vi "Handle Error.vi"(8 "error in (no error)":errorcluster caption="错误输入（无错误）", 11 "ErrorHanlder in":refnum<class "ErrorHanlder.lvclass"> caption="操作者输入") -> (0 "error out":errorcluster caption="错误输出", 2 "stop actor?":bool=TRUE caption="停止操作者？", 3 "ErrorHanlder out":refnum<class "ErrorHanlder.lvclass"> caption="操作者输出")   [LabVIEW 2019, in "ErrorHanlder.lvlib" / "ErrorHanlder.lvclass"]
doc: "(<B>Filename</B>: Actor Framework.lvlib:Actor.lvclass:Handle Error.vi)\n\nDefines how the actor handles an error that occurred while processing a message.默认情况下，该方法不执行任何操作，仅停止操作者。"
uses:
  ErrorHanlder.lvclass
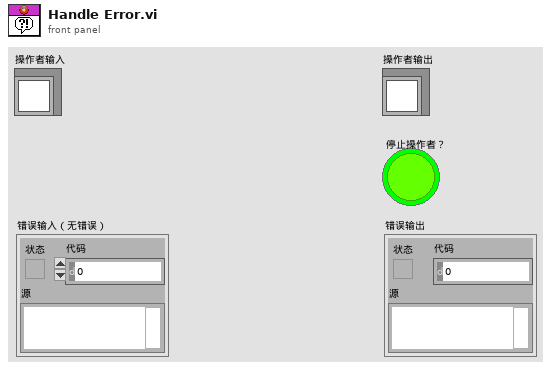
[diagram p1: front panel]
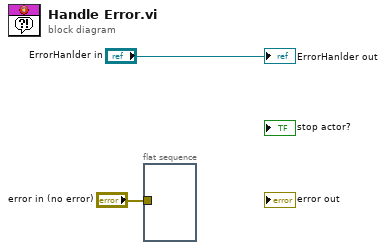
[diagram p0: block diagram]
diagram:
  n1 = flat-sequence {
    tunnel: "error in (no error)" -> [_]
    frame #0 {
    }
  }
  "ErrorHanlder out" <- "ErrorHanlder in"
